vi "Init USB_TC.vi"(8 "error in":errorcluster) -> (0 "error out":errorcluster, 3 "task out":refnum<k21>)   [LabVIEW 2018]
uses:
  <vilib>/DAQmx/create/channels.llb/DAQmx Create Channel (AI-Temperature-Thermocouple).vi
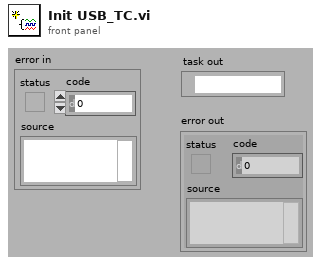
[diagram p1: front panel]
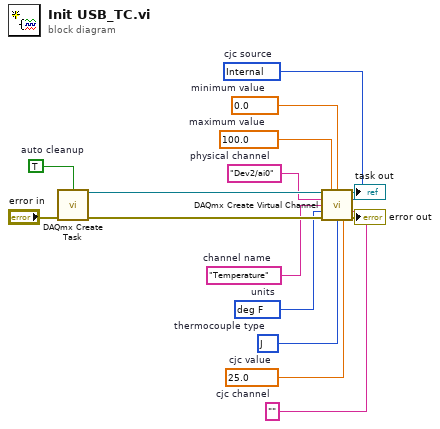
[diagram p0: block diagram]
diagram:
  w2 = ""  # cjc channel
  w3 = u32 10200 items=["Internal"=10200, "Constant Value"=10116, "Channel"=10113]  # cjc source
  w4 = 25.0  # cjc value
  w5 = 10072 items=["J"=10072, "K"=10073, "N"=10077, "R"=10082, "S"=10085, "T"=10086, "B"=10047, "E"=10055]  # thermocouple type
  w6 = 10144 items=["deg C"=10143, "deg F"=10144, "Kelvins"=10325, "deg R"=10145, "From Custom Scale"=10065]  # units
  w1 = "Temperature"  # channel name
  w9 = 0.0  # minimum value
  w10 = 100.0  # maximum value
  w11 = "Dev2/ai0"  # physical channel
  w13 = TRUE  # auto cleanup
  n1 = call <vilib>:"DAQmx Create Task.vi"("auto cleanup"=w13, "error in"="error in") -> ("task out"=w12:refnum<k21>, "error out"=w14:errorcluster)  [unwired: 12 in]
  n2 = call-poly <vilib>:"DAQmx Create Virtual Channel.vi"("task in"=w12, "maximum value"=w10, "minimum value"=w9, "physical channels"=w11, "cjc source"=w3, "name to assign"=w1, "units"=w6, "cjc channel"=w2, "error in"=w14, "thermocouple type"=w5, "cjc value"=w4) -> ("task out"=→"task out":refnum<k21>, "error out"=→"error out":errorcluster)  [unwired: 3 in]
